vi "LWXPS_GetJogAcceleration.vi"(1 "XPS Reference IN":refnum<k24>, 4 "LabVIEW error IN":errorcluster) -> (12 "XPS Reference OUT":refnum<k24>, 13 "LabVIEW error OUT":errorcluster, 14 "Returned error code":i32, 15 "X Acceleration time ( ms )":i32, 16 "X Smooth factor ( ms )":i32, 17 "Y Acceleration time ( ms )":i32, 18 "Y Smooth factor ( ms )":i32, 19 "XPS Error String":string)   [LabVIEW 2014]
uses:
  D:/XPSQ8_LabView_Library/Development/Source/Dll/Newport.XPS.CommandInterface.dll
  Dll/Newport.XPS.CommandInterface.dll
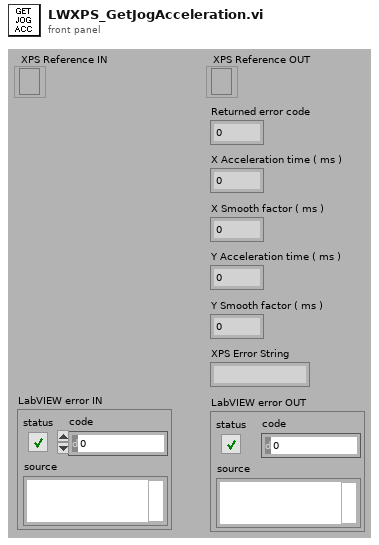
[diagram p1: front panel]
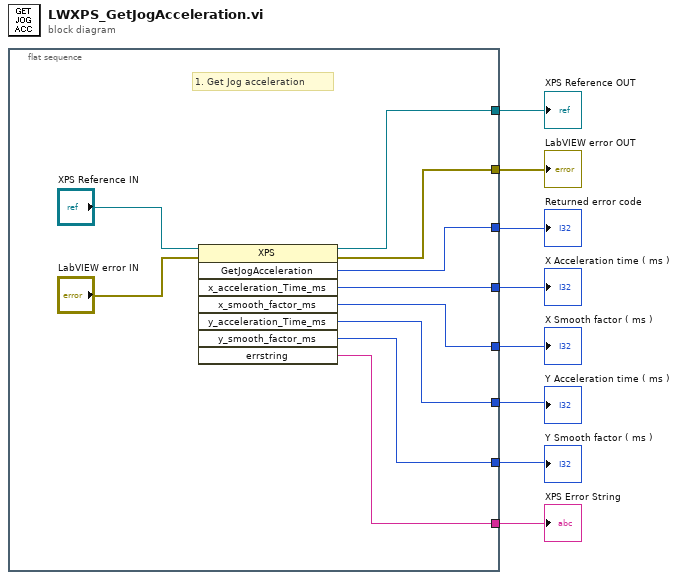
[diagram p0: block diagram]
diagram:
  n1 = flat-sequence {
    tunnel: [w17] -> w8
    tunnel: [w16] -> w7
    tunnel: [w15] -> w6
    tunnel: [w13] -> w5
    tunnel: [w12] -> w4
    tunnel: [w11] -> w3
    tunnel: [w10] -> w2
    tunnel: [w9] -> w1
    frame #0 {
      # "1. Get Jog acceleration"
      n2 = invoke class="XPS" method="GetJogAcceleration"(reference="XPS Reference IN", error in="LabVIEW error IN") -> (reference out=w17:refnum<k24>, error out=w16:errorcluster, "GetJogAcceleration"=w15:i32, "x_acceleration_Time_ms"=w13:i32, "x_smooth_factor_ms"=w12:i32, "y_acceleration_Time_ms"=w11:i32, "y_smooth_factor_ms"=w10:i32, "errstring"=w9:string)  [unwired: 6 in]
    }
  }
  "XPS Reference OUT" <- w8
  "LabVIEW error OUT" <- w7
  "Returned error code" <- w6
  "X Acceleration time ( ms )" <- w5
  "X Smooth factor ( ms )" <- w4
  "Y Acceleration time ( ms )" <- w3
  "Y Smooth factor ( ms )" <- w2
  "XPS Error String" <- w1
